vi "toSlashCodeString.vi"(8 "error in (no error)":errorcluster, 11 "String In":string) -> (0 "error out":errorcluster, 3 "String Out":string)   [LabVIEW 2013, in "BSON.lvlib"]
uses:
  BSON.lvlib
  <vilib>/regexp/Match Regular Expression.xnode
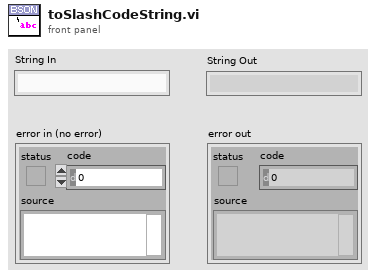
[diagram p1: front panel]
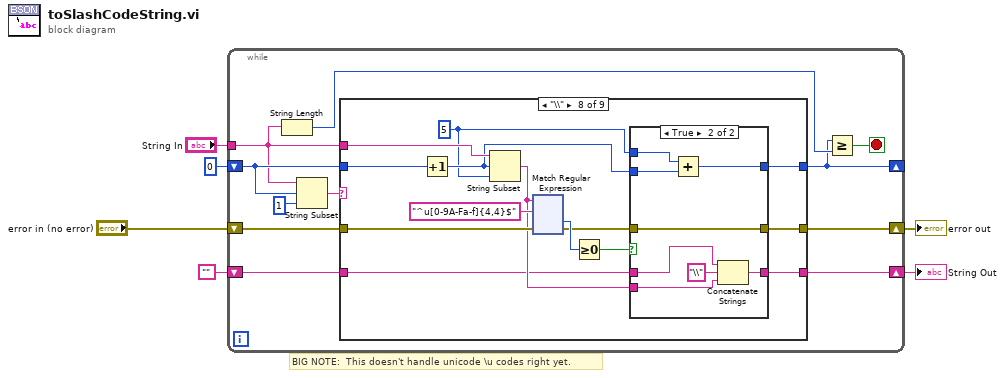
[diagram p0: block diagram]
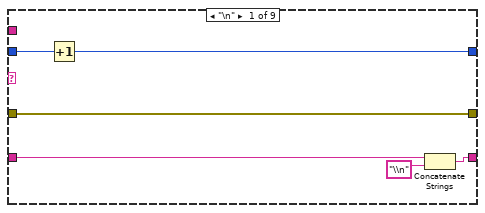
[diagram p2: hidden frame]
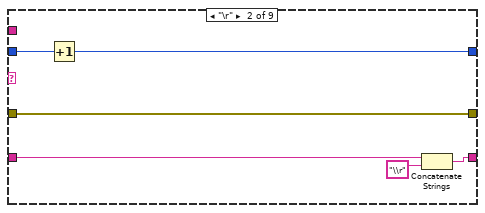
[diagram p3: hidden frame]
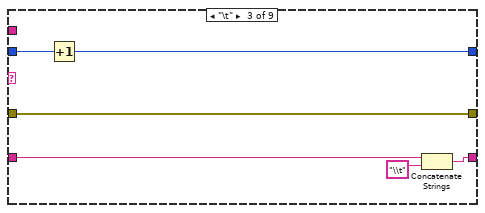
[diagram p4: hidden frame]
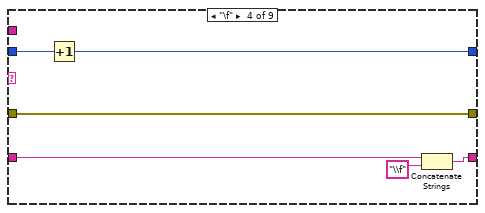
[diagram p5: hidden frame]
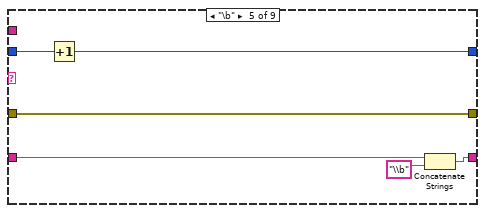
[diagram p6: hidden frame]
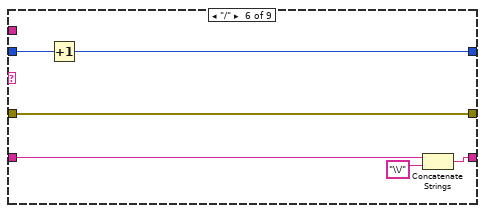
[diagram p7: hidden frame]
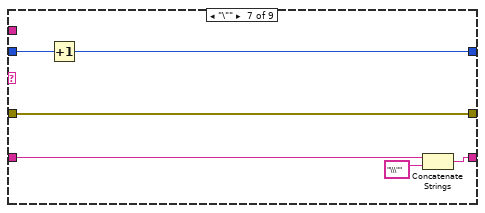
[diagram p8: hidden frame]
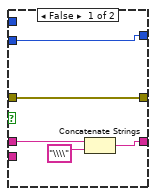
[diagram p9: hidden frame]
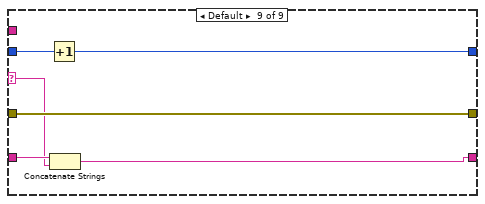
[diagram p10: hidden frame]
diagram:
  # "BIG NOTE:  This doesn't handle unicode \\u codes right yet."
  n1 = while {
    shift-right: [w11] -> w6
    shift-left: "error in (no error)" -> [w15]
    tunnel: "String In" -> [w9]
    shift-right: [w13] -> w1
    shift-left: "" -> [w14]
    shift-right: [w7] -> _
    shift-left: 0 -> [w12]
    stop <- w10 stop-if-true
    n2 = String Length(string=w9) -> (length=w8:i32)
    n3 = String Subset(string=w9, offset (0)=w12, length (rest)=1 ("length (rest)")) -> (substring=w16:string)
    n4 = case shown="\"\\\\\"" w16 {
      selector: w16 -> [_ _ _ _ _ _ _ _ w199]
      tunnel: w15 -> [w18 w25 w31 w37 w43 w49 w55 w71 w201]
      tunnel: w14 -> [w23 w29 w35 w41 w47 w53 w59 w60 w200]
      tunnel: [w22 w28 w34 w40 w46 w52 w58 w65 w198] -> w13
      tunnel: w12 -> [w20 w27 w33 w39 w45 w51 w57 w73 w203]
      tunnel: [w19 w26 w32 w38 w44 w50 w56 w62 w202] -> w7
      tunnel: [w18 w25 w31 w37 w43 w49 w55 w64 w201] -> w11
      tunnel: w9 -> [_ _ _ _ _ _ _ w72 _]
      frame "\n" {
        n5 = Increment(x=w20) -> (x+1=w19:i32)
        n6 = Concatenate Strings(w23, "\\n") -> (w22:string)
      }
      frame "\r" {
        n7 = Increment(x=w27) -> (x+1=w26:i32)
        n8 = Concatenate Strings(w29, "\\r") -> (w28:string)
      }
      frame "\t" {
        n9 = Increment(x=w33) -> (x+1=w32:i32)
        n10 = Concatenate Strings(w35, "\\t") -> (w34:string)
      }
      frame "\f" {
        n11 = Increment(x=w39) -> (x+1=w38:i32)
        n12 = Concatenate Strings(w41, "\\f") -> (w40:string)
      }
      frame "\b" {
        n13 = Increment(x=w45) -> (x+1=w44:i32)
        n14 = Concatenate Strings(w47, "\\b") -> (w46:string)
      }
      frame "/" {
        n15 = Increment(x=w51) -> (x+1=w50:i32)
        n16 = Concatenate Strings(w53, "\\/") -> (w52:string)
      }
      frame "\"" {
        n17 = Increment(x=w57) -> (x+1=w56:i32)
        n18 = Concatenate Strings(w59, "\\\"") -> (w58:string)
      }
      frame "\\" {
        w61 = 5 ("length (rest)")
        n19 = Increment(x=w73) -> (x+1=w63:i32)
        n20 = String Subset(string=w72, offset (0)=w63, length (rest)=w61) -> (substring=w66:string)
        n21 = xnode "Match Regular Expression"("input string"=w66, "regular expression"="^u[0-9A-Fa-f]{4,4}$", "error in"=w71) -> ("offset past match"=w69:i32, "error out"=w68:errorcluster)  [unwired: 3 in, 3 out]
        n22 = Greater Or Equal To 0?(x=w69) -> (x >= 0?=w67:bool)
        n23 = case shown="True" w67 {
          tunnel: w68 -> [w78 w86]
          tunnel: w66 -> [_ w80]
          tunnel: [w76 w82] -> w65
          tunnel: [w78 w86] -> w64
          tunnel: w63 -> [w77 w85]
          tunnel: [w77 w83] -> w62
          tunnel: w61 -> [_ w84]
          tunnel: w60 -> [w75 w81]
          frame False {
            n24 = Concatenate Strings(w75, "\\\\" ("string")) -> (w76:string)
          }
          frame True {
            n25 = Add(x=w84, y=w85) -> (x+y=w83:i32)
            n26 = Concatenate Strings(w81, "\\" ("string"), w80) -> (w82:string)
          }
        }
      }
      frame Default {
        n27 = Increment(x=w203) -> (x+1=w202:i32)
        n28 = Concatenate Strings(w200, w199) -> (w198:string)
      }
    }
    n29 = Greater Or Equal?(x=w7, y=w8) -> (x >= y?=w10:bool)
  }
  "String Out" <- w1
  "error out" <- w6
